vi "MQTT_SubAck_Read.vi"(8 "error in (no error)":errorcluster, 11 "connection ID":refnum<k5>) -> (0 "error out":errorcluster, 1 "Granted QoS Levels":T1(array[ring]), 3 "connection ID out":refnum<k5>)   [LabVIEW 2025, in "DAQIO MQTT.lvlib"]
doc: "© 2015 - daq.io, LLC - Peter Adelhardt"
uses:
  DAQIO MQTT.lvlib
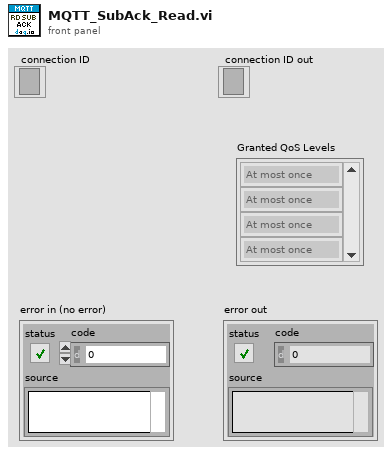
[diagram p1: front panel]
types:
  T1 = enum8{"At most once", "At least once", "Exactly once", "Reserved"}[]
  T2 = enum8{"At most once", "At least once", "Exactly once", "Reserved"}
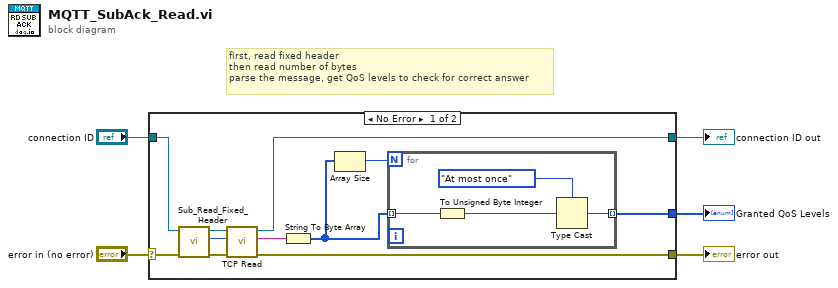
[diagram p0: block diagram]
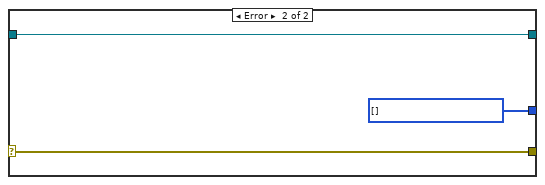
[diagram p2: hidden frame]
diagram:
  # "first, read fixed header\nthen read number of bytes\nparse the message, get QoS levels to check for correct answer"
  n1 = case shown="No Error" "error in (no error)" {
    selector: "error in (no error)" -> [w12 w23]
    tunnel: [w10 w23] -> w4
    tunnel: [w8 w22] -> w3
    tunnel: [w7 w21] -> w2
    tunnel: "connection ID" -> [w6 w21]
    frame No Error {
      n2 = call "Sub_Read_Fixed_Header.vi"("error in (no error)"=w12, "connection ID"=w6) -> ("error out"=w11:errorcluster, "Remaining Length"=w14:u32, "connection ID out"=w13:refnum<k5>)  [unwired: 3 in, 4 out]
      n3 = call "TCP Read.vi"("error in (no error)"=w11, "bytes to read"=w14, "connection ID"=w13) -> ("error out"=w10:errorcluster, "data out"=w15:string, "connection ID out"=w7:refnum<k5>)  [unwired: 6 in]
      n4 = String To Byte Array(string=w15) -> (unsigned byte array=w9:u8[])
      n5 = Array Size(array=w9) -> (size(s)=w16:i32)
      n6 = for {
        N: w16 -> [_]
        tunnel: [w19] -> w8 mode=indexing
        tunnel: w9 -> [w18] mode=indexing
        n7 = To Unsigned Byte Integer(number=w18) -> (unsigned 8bit integer=w17:u8)
        n8 = Type Cast(type=T2."At most once" ("QoS Level"), x=w17) -> (*(type *) &x=w19:T2)
      }
    }
    frame Error {
      w22 = T1 [] items=["At most once", "At least once", "Exactly once", "Reserved"]
    }
  }
  "error out" <- w4
  "Granted QoS Levels" <- w3
  "connection ID out" <- w2
